vi "Menu - Get Checked State.vi"(8 "error in (no error)":errorcluster, 10 "item tag":string, 11 "menu reference":refnum<k9>) -> (0 "error out":errorcluster, 3 "checked":bool)   [LabVIEW 2015]
doc: "Returns the Checked? propert of the desired menu item."
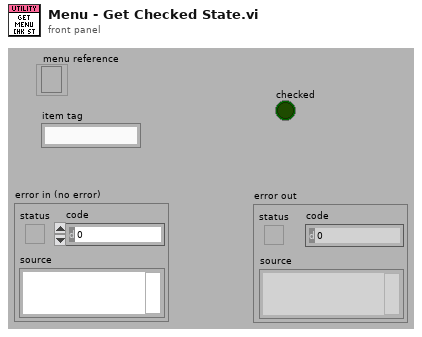
[diagram p1: front panel]
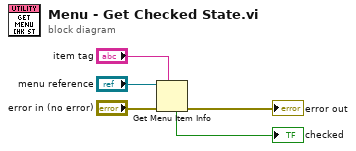
[diagram p0: block diagram]
diagram:
  n1 = Get Menu Item Info(7:"item tag", 8:"error in (no error)", 11:"menu reference") -> (0:→"error out":errorcluster, 4:→"checked":bool)  [unwired: 5 out]
